vi "GetProjectFromProjectPath.vi"(8 "Fehler (Eingang, kein Fehler)":errorcluster, 11 "ProjectPfad":path) -> (0 "Fehler (Ausgang)":errorcluster, 3 "Projekt Referenz":refnum<vi>)   [LabVIEW 2020, in "ConditionalDeactivation.lvlib"]
doc: "For PreBuildAction to find the actual Project (for conditional deactivaion values - different context !)\n\nriw, 10.03.2020"
uses:
  ConditionalDeactivation.lvlib
panel:
  out "Name":string
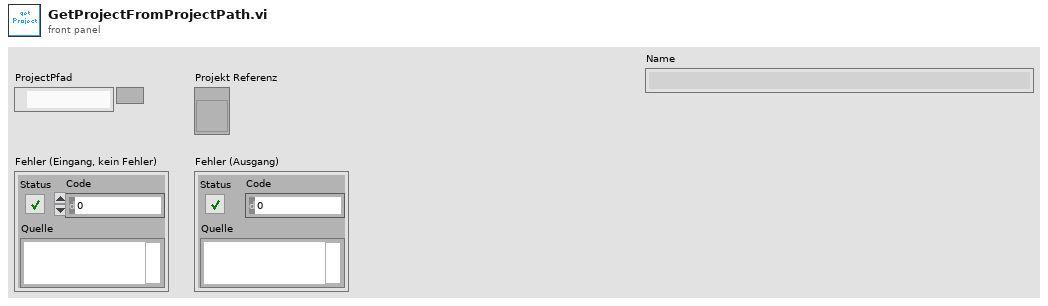
[diagram p1: front panel]
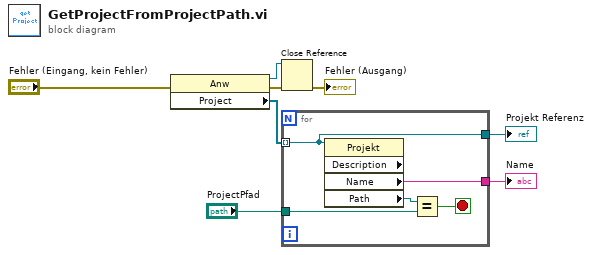
[diagram p0: block diagram]
diagram:
  n1 = property class="Anw"(error in="Fehler (Eingang, kein Fehler)") -> (reference out=w3:refnum<vi>, error out=w2:errorcluster, "Project"=w8:refnum<vi>[])  [unwired: 1 in]
  n2 = Close Reference(reference=w3, error in (no error)=w2) -> (error out=→"Fehler (Ausgang)":errorcluster)
  n3 = for {
    tunnel: w8 -> [w10] mode=indexing
    tunnel: "ProjectPfad" -> [w12]
    tunnel: [w11] -> w5
    tunnel: [w10] -> w6
    stop <- w9 stop-if-true
    n4 = property class="Projekt" props=["Description", "Name", "Path"](reference=w10) -> ("Name"=w11:string, "Path"=w13:path)  [unwired: 1 in, 3 out]
    n5 = Equal?(x=w13, y=w12) -> (x = y?=w9:bool)
  }
  "Projekt Referenz" <- w6
  "Name" <- w5
